vi "testrotation.vi"() -> ()   [LabVIEW 2022 SP3]
uses:
  C:/Users/Public/OneDrive/Desktop/PMT program/SampleCodeLabView/Kinesis_with_LabVIEW_Examples_LV12 - v3/Thorlabs.MotionControl.Controls.dll
  C:/Users/Public/OneDrive/Desktop/PMT program/SampleCodeLabView/Kinesis_with_LabVIEW_Examples_LV12 - v3/ThorLabs.MotionControl.KCube.DCServoCLI.dll
panel:
  out "PC":dbl caption="Current Rotation Position"
  in  "quarter waveplate p2":dbl=221.0 format="%#_13g"
  in  "quarter waveplate p1":dbl=131.0 format="%#_13g"
  in  "Motor Controller\nSerialNumber":string="27268499"
  in  "KCubeDCServoControl":refnum<k24>(container)
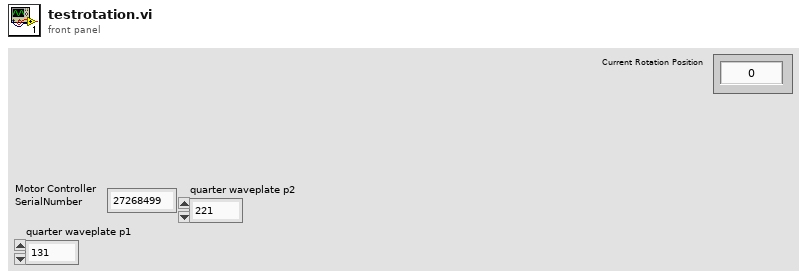
[diagram p1: front panel]
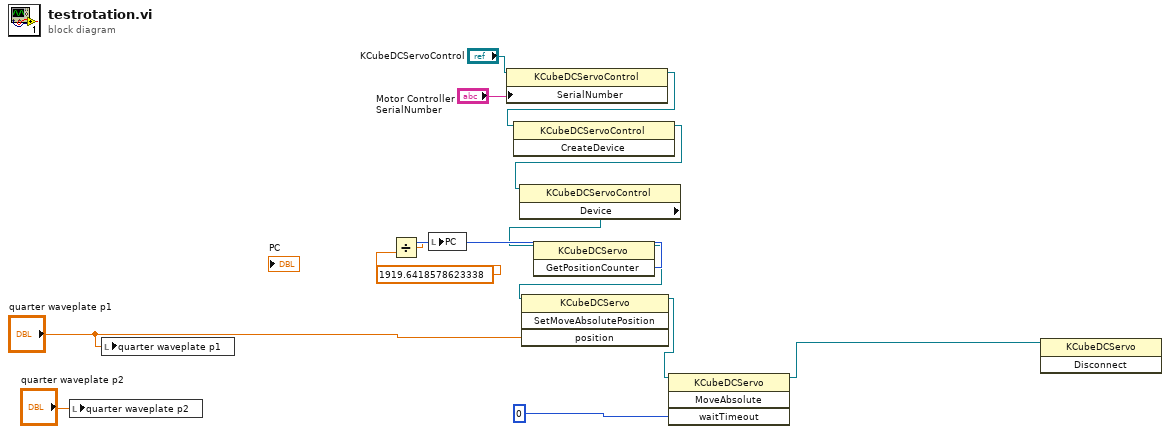
[diagram p0: block diagram]
diagram:
  n1 = local write "quarter waveplate p2"("quarter waveplate p2") -> ()
  n2 = local write "quarter waveplate p1"("quarter waveplate p1") -> ()
  n3 = property class="KCubeDCServoControl"(reference="KCubeDCServoControl", "SerialNumber"="Motor Controller\nSerialNumber") -> (reference out=w3:refnum<k24>)  [unwired: 1 in, 1 out]
  n4 = invoke class="KCubeDCServoControl" method="CreateDevice"(reference=w3) -> (reference out=w4:refnum<k24>)  [unwired: 2 in, 2 out]
  n5 = property class="KCubeDCServoControl"(reference=w4) -> ("Device"=w2:refnum<k24>)  [unwired: 1 in, 2 out]
  n6 = invoke class="KCubeDCServo" method="GetPositionCounter"(reference=w2) -> (reference out=w9:refnum<k24>, "GetPositionCounter"=w12:i32)  [unwired: 2 in, 1 out]
  n7 = Divide(x=w12, y=1919.6418578623338) -> (x/y=w10:dbl)
  n8 = local write "PC"(w10) -> ()
  n9 = invoke class="KCubeDCServo" method="SetMoveAbsolutePosition"(reference=w9, "position"="quarter waveplate p1") -> (reference out=w5:refnum<k24>)  [unwired: 2 in, 3 out]
  n10 = invoke class="KCubeDCServo" method="MoveAbsolute"(reference=w5, "waitTimeout"=0) -> (reference out=w1:refnum<k24>)  [unwired: 2 in, 3 out]
  n11 = invoke class="KCubeDCServo" method="Disconnect"(reference=w1) -> ()  [unwired: 2 in, 3 out]
